vi "OnProcessRequest.vi"(4 "User Parameter":variant, 5 "Event Data":cluster{"sender":refnum<k24>, "e":refnum<k24>}, 6 "Control Ref":refnum<k24>, 7 "Event Common Data":T1) -> ()   [LabVIEW 2013]
uses:
  E:/Dropbox/ni/lvcef/github/lvcef/dotnet/LVCef/bin/Debug/LVCef.dll
  dotnet/LVCef/bin/Debug/LVCef.dll
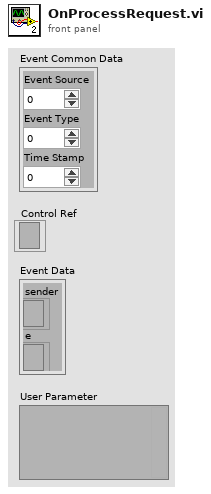
[diagram p1: front panel]
types:
  T1 = cluster{"Event Source":i32, "Event Type":u32, "Time Stamp":u32}
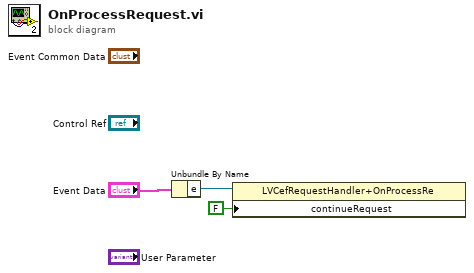
[diagram p0: block diagram]
diagram:
  n1 = Unbundle By Name("Event Data") -> ("e"=w2:refnum<k24>)
  n2 = property class="LVCefRequestHandler+OnProcessRe"(reference=w2, "continueRequest"=FALSE) -> ()  [unwired: 1 in, 2 out]
